vi "BIO_free.vi"(8 "error in (no error)":errorcluster, 11 "BIO in":refnum<class "BIO.lvclass">) -> (0 "error out":errorcluster, 2 "return type":i32)   [LabVIEW 2013, in "OpenSSL Socket.lvlib" / "BIO.lvclass"]
uses:
  BIO.lvclass
  SSL-Lib/SSL-Lib.lvclass/SSL-Lib.ctl
  BIO.lvclass/BIO.ctl
  SSL-Lib/Read Crypto Library Path.vi
  Read Handle.vi
  SSL-Lib/SSL-Lib.lvclass
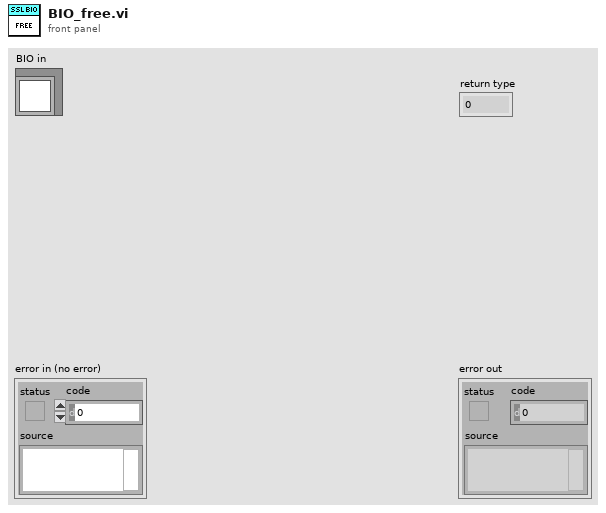
[diagram p1: front panel]
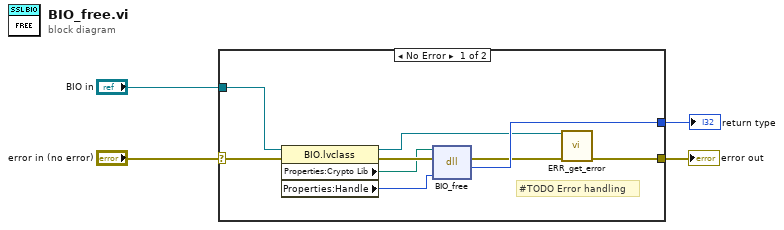
[diagram p0: block diagram]
diagram:
  n1 = case shown="No Error" "error in (no error)" {
    selector: "error in (no error)" -> [w13 w14]
    tunnel: [w6 w14] -> w3
    tunnel: "BIO in" -> [w8 _]
    tunnel: [w12 _] -> w1
    frame No Error {
      # "#TODO Error handling"
      n2 = property class="BIO.lvclass"(reference=w8, error in=w13) -> (reference out=w5:refnum<class "BIO.lvclass">, error out=w11:errorcluster, "Properties:Crypto Lib"=w9:path, "Properties:Handle"=w10:u64)
      n3 = dll-call lib="C:/Program Files (x86)/National Instruments/Shared/nissl/NIlibeay32.dll" fn="BIO_free"(path in=w9, error in=w11, "BIO"=w10) -> (error out=w7:errorcluster, "return type"=w12:i32)  [unwired: 2 in, 1 out]
      n4 = call "ERR_get_error.vi"("error in (no error)"=w7, "SSL-Lib in"=w5) -> ("error out"=w6:errorcluster)  [unwired: 8 in, 1 out]
    }
    frame Error {
    }
  }
  "error out" <- w3
  "return type" <- w1
